vi "Get Node Type.vi"(8 "error in":errorcluster, 11 "Node in":refnum<class "Node.lvclass">) -> (0 "error out":errorcluster, 3 "Node out":refnum<class "Node.lvclass">)   [LabVIEW 2014, in "Node.lvclass"]
uses:
  Node.lvclass
  <resource>/objmgr/DOMUserDefRef.rc
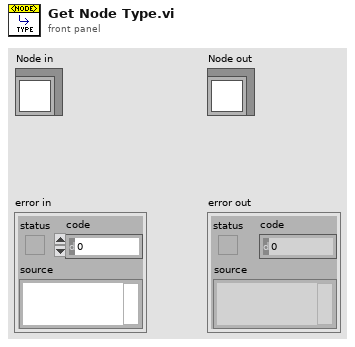
[diagram p1: front panel]
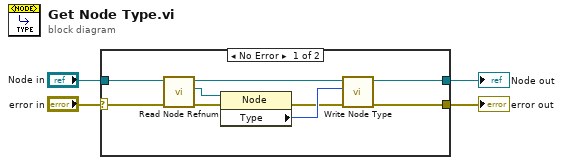
[diagram p0: block diagram]
diagram:
  n1 = case shown="No Error" "error in" {
    selector: "error in" -> [w6 w15]
    tunnel: [w5 w15] -> w3
    tunnel: [w10 w14] -> w1
    tunnel: "Node in" -> [w13 w14]
    frame No Error {
      n2 = call-dynamic "Read Node Refnum.vi"("error in"=w6, "Node in"=w13) -> ("error out"=w8:errorcluster, "Node Refnum"=w11:refnum<k20>, "Node out"=w12:refnum<class "Node.lvclass">)  [unwired: 7 in]
      n3 = property class="Node"(reference=w11, error in=w8) -> (error out=w7:errorcluster, "Type"=w9:i32)  [unwired: 1 out]
      n4 = call-dynamic "Write Node Type.vi"("error in"=w7, "Node Type"=w9, "Node in"=w12) -> ("error out"=w5:errorcluster, "Node out"=w10:refnum<class "Node.lvclass">)  [unwired: 7 in]
    }
    frame Error {
    }
  }
  "error out" <- w3
  "Node out" <- w1
